vi "helicopter.vi"() -> ()   [LabVIEW 2017]
uses:
  controls/state.ctl
  controls/arrays and heights.ctl
  controls/scores.ctl
  <vilib>/sound2/lvsound2.llb/Sound Output Task ID.ctl
  <vilib>/sound2/lvsound2.llb/Sound Output Set Volume (Single).vi
panel:
  out "Waveform Chart":waveform(dbl)[](graph)=[{"t0"=timestamp(75 s since 1904-01-01), "dt"=1.0, "Y"=[90.36613236635097, 90.06036176170126, 89.42608442122003, 89.31247150775786, 88.85183588729195, 88.07425750121689, 88.69261658515198, 87.86425557558843, 88.68598594735637, 89.37218640366484, 88.87909011717896, 89.2723214289112, 89.37198808916769, 89.3075761436066, 89.59339067781413, 89.09888409349647, 89.89015333376268, 89.02148210217948, 89.47099401182557, 89.25048133248812, 89.38897358327958, 89.77746190833348, 90.53755429906346, 91.28574771023173, 90.94907051126542, 90.31859843418972, 90.86724841965984, 90.63431666280458, 91.36203841742443, 92.04622343431689, 91.2238317034208, 90.39079136550929, 89.84037866388954, 89.6430353390771, 90.19775011068187, 89.34296034585601, 88.87882107659819, 88.68974069015621, 89.40076042601159, 88.75168446743764, 87.95702372899578, 88.65736922287022, 87.90799712470135, 87.54405824486757, 87.74580039145059, 87.72021014407412, 87.91110658053051, 88.72125981331965, 88.50217712958094, 88.66901306015122, 88.44710332072938, 89.2439046034086, 89.44541276476619, 89.49348158640845, 90.23930384605846, 90.77006534815207, 91.56141906157212, 92.1965278095345, 91.61779502995512, 91.68953912575036, 91.7353123580429, 91.13420107041388, 91.29336740149286, 91.62246065547052, 92.32580838508346, 92.94681638984402, 93.63800419438708, 94.43512822801334, 95.09729030042807, 94.89218320830427, 95.29402122869416, 95.18981755244249, 94.53360430397686, 94.27656624709857, 94.95521955315563, 95.75593296599362, 95.13068608073014, 95.87345050233536, 96.41159434256669, 97.01259955208491, 96.59292222657096, 95.89637511486526, 96.58985501237102, 97.18611274172392, 97.70234591984999, 97.33615669802494, 96.72130798541049, 97.44479281384942, 97.84458360370694, 96.99411772170845, 97.83904016371078, 98.54327276615516, 98.84951280333539, 99.26520954670279, 99.7106233231448, 98.89367163173466, 98.55486364541227, 98.33140165697876, 97.47445939153363, 96.91169513152757, 96.77239204274291]}, {"t0"=timestamp(0 s since 1904-01-01), "dt"=1.0, "Y"=[50.0, 50.0, 50.0, 50.0, 50.0, 50.0, 50.0, 50.0, 50.0, 50.0, 50.0, 50.0, 50.0, 50.0, 50.0, 50.0, 50.0, 50.0, 50.0, 50.0, 50.0, 50.0, 50.0, 50.0, 50.0, 50.0, 50.0, 50.0, 50.0, 50.0, 50.0, 50.0, 50.0, 50.0, 50.0, 50.0, 50.0, 49.963212500000004, 49.901900000000005, 49.81606250000001, 49.70570000000001, 49.57081250000001, 49.41140000000001, 49.22746250000001, 49.01900000000001, 48.78601250000001, 48.528500000000015, 48.246462500000014, 47.939900000000016, 47.60881250000002, 47.25320000000002, 46.873062500000024, 46.47777500000002, 46.07358750000002, 45.66675000000002, 45.26351250000002, 44.87012500000002, 44.49283750000002, 44.13790000000002, 43.81156250000002, 43.52007500000002, 43.269687500000025, 43.066650000000024, 42.917212500000026, 42.827625000000026, 42.804137500000024, 42.85300000000002, 42.98046250000002, 43.192490909090935, 43.48605492424245, 43.861154545454575, 44.3177897727273, 44.85596060606064, 45.475667045454585, 46.176909090909135, 46.95968674242429, 47.82400000000005, 48.76984886363641, 49.79723333333339, 50.90615340909097, 52.096609090909155, 53.368600378787946, 54.72212727272734, 56.15718977272734, 57.67378787878795, 59.26254659090916, 60.91721590909098, 62.6315458333334, 64.39928636363643, 66.21418750000008, 68.06999924242433, 69.96047159090918, 71.87935454545463, 73.8203981060607, 75.77735227272736, 77.74396704545464, 79.7139924242425, 81.68117840909099, 83.63927500000008, 85.58203219696978, 87.50320000000009]}, {"t0"=timestamp(75 s since 1904-01-01), "dt"=1.0, "Y"=[5.832101008474922, 5.159278583421013, 5.801309156356126, 6.28595492791603, 6.165150175868025, 5.391838078029318, 5.660821421593425, 6.290693171535654, 5.486359312466074, 4.980595454428121, 5.743102722515479, 5.30778379381289, 5.55585812403333, 4.705780686732893, 5.2333896609954405, 4.963823736280907, 5.822464417498429, 6.642853398607047, 6.668353285980142, 6.089309556691314, 6.609858622855841, 5.982411212743665, 5.438514421617222, 6.263955715844029, 5.531193565870151, 5.801494600625852, 5.566031242846543, 5.115602472848708, 4.8481344780389595, 5.442184030722513, 5.149905285075606, 5.323279727659692, 5.065894282439003, 5.104924163660315, 4.891177011196872, 4.93812604547638, 5.067990838692791, 4.41324137869173, 3.5767367766417517, 2.792679923924744, 2.4382317997087983, 2.671144146629132, 3.1776714395653554, 3.690271474648958, 3.367994065506265, 3.215178406627257, 3.569049632721444, 3.463406971992561, 3.3200051907081365, 3.725695826201605, 3.0566988241284543, 3.4748166261830487, 2.879357702129107, 3.258851993085851, 2.522144166423153, 3.1542111118236003, 3.5230799629696405, 3.9745896259951596, 4.195366575820299, 4.883766157691795, 4.662673212944459, 5.034075317396015, 5.473994783784907, 4.699819872968005, 4.061002012703361, 3.197689491225556, 2.927623166451658, 3.7805700044544763, 3.210549827499141, 3.411153283350134, 2.6885766219340868, 3.4848113994331325, 3.8765381933384324, 3.565085003146204, 4.2186698007162295, 4.443019252189356, 4.859586669337306, 5.307331570893703, 4.60484270830926, 4.8982383059707155, 4.805761589310327, 4.454111165255858, 5.024113691840286, 4.881538126174325, 5.292346594076474, 5.233885183603672, 5.771407868577864, 5.6442442129488715, 6.45349714065848, 6.326226502898815, 5.886373600897694, 6.685385577016143, 7.325174833405951, 7.254372612866276, 7.680755742430742, 7.701210685658931, 7.8289177080882535, 8.447237862350994, 8.214394126067315, 8.955412687632835, 9.120288920602299]}, {"t0"=timestamp(75 s since 1904-01-01), "dt"=1.0, "Y"=[-150.0, -150.0, -150.0, -150.0, -150.0, -150.0, -150.0, -150.0, -150.0, -150.0, -150.0, -150.0, -150.0, -150.0, -150.0, -150.0, -150.0, -150.0, -150.0, -150.0, -150.0, -150.0, -150.0, -150.0, -150.0, -150.0, -150.0, -150.0, -150.0, -150.0, -150.0, -150.0, -150.0, -150.0, -150.0, -150.0, -150.0, -150.0, -150.0, -150.0, -150.0, -150.0, -150.0, -150.0, -150.0, -150.0, 150.0, 150.0, 150.0, 150.0, 150.0, 150.0, 150.0, 150.0, 150.0, 150.0, 38.0, 38.0, 38.0, 38.0, 38.0, 38.0, 38.0, 38.0, 38.0, 38.0, -38.0, -38.0, -38.0, -38.0, -38.0, -38.0, -38.0, -38.0, -38.0, -38.0, 5.0, 5.0, 5.0, 5.0, 5.0, 5.0, 5.0, 5.0, 5.0, 5.0, -5.0, -5.0, -5.0, -5.0, -5.0, -5.0, -5.0, -5.0, -5.0, -5.0, 9.0, 9.0, 9.0, 9.0, 9.0]}]
  in  "View High Scores":bool
  in  "Music?":bool
  out "Score":dbl=132.0 format="%#.12g"
  in  "Difficulty":enum16{"Easy", "Normal", "Hard"}(ring)=enum."Normal"
  out "Acceleration (m/s^2)":dbl(knob)=-7.385757575757571 scale=-10.0..10.0
  in  "Cancel Button":bool
  in  "Start":bool
  out "Fuel (L)":dbl(knob)=150.0 scale=0.0..300.0
  in  "Thrust (m/s^2)":dbl(slide)=21.212121212121215 scale=0.0..50.0
  in  "Vertical Thrusters!":bool
  out "Large Helicopter Image":u8[][](graph)
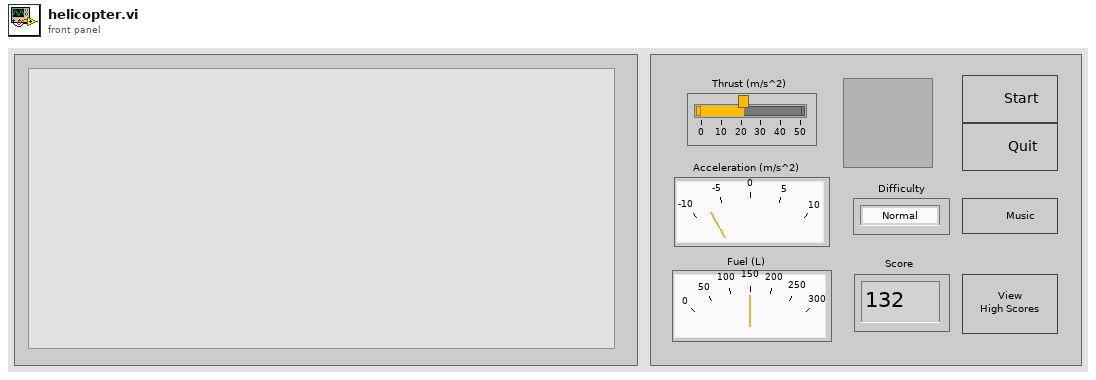
[diagram p1: front panel]
types:
  T1 = typedef "Sound Output Task ID.ctl" = u32
  T2 = typedef "arrays and heights.ctl" = cluster{"Score Array":T3[], "Lowest high score":dbl, "Score":dbl, "Ceiling":dbl, "Floor":dbl, "Ceiling Array":dbl[], "Floor array":dbl[], "Helicopter height":dbl, "Helicopter array":dbl[], "Fuel":dbl, "Fuel array":dbl[], "fuel counter":i32, "obstacle counter":i32, "Obstacle array":dbl[], "helicopter v_0":dbl, "helicopter a_0":dbl, "Obstacle height":dbl}
  T3 = typedef "scores.ctl" = cluster{"Score":dbl, "Name":string, "Date":string}
  T4 = typedef "state.ctl" = enum16{"Wait", "Init", "Run", "Death", "Write High Score", "View High Scores", "Difficulty", "Stop"}
  T5 = typedef "game parameters.ctl" = cluster{"Upper Limit (m)":dbl, "Lower Limit (m)":dbl, "Obstacle time":dbl, "Obstacle length":dbl, "fuel decrement":dbl, "Fuel time":dbl, "fuel amount":dbl, "Fuel range":i32, "Death range":i32, "Terrain slope":dbl, "Speed (km/hr)":dbl, "Time step (ms)":u32, "Gravity":dbl, "Date":string, "High scores path":path, "Difficulty":enum16{"Easy", "Normal", "Hard"}, "Headstart":u32}
  T6 = typedef "Sound Paths.ctl" = cluster{"Crash sound path":path, "Music path":path, "Thrust sound path":path, "High score sound path":path}
  T7 = typedef "image arrays.ctl" = cluster{"Helicopter image":u8[][], "Flame image":u8[][], "Large image":u8[][]}
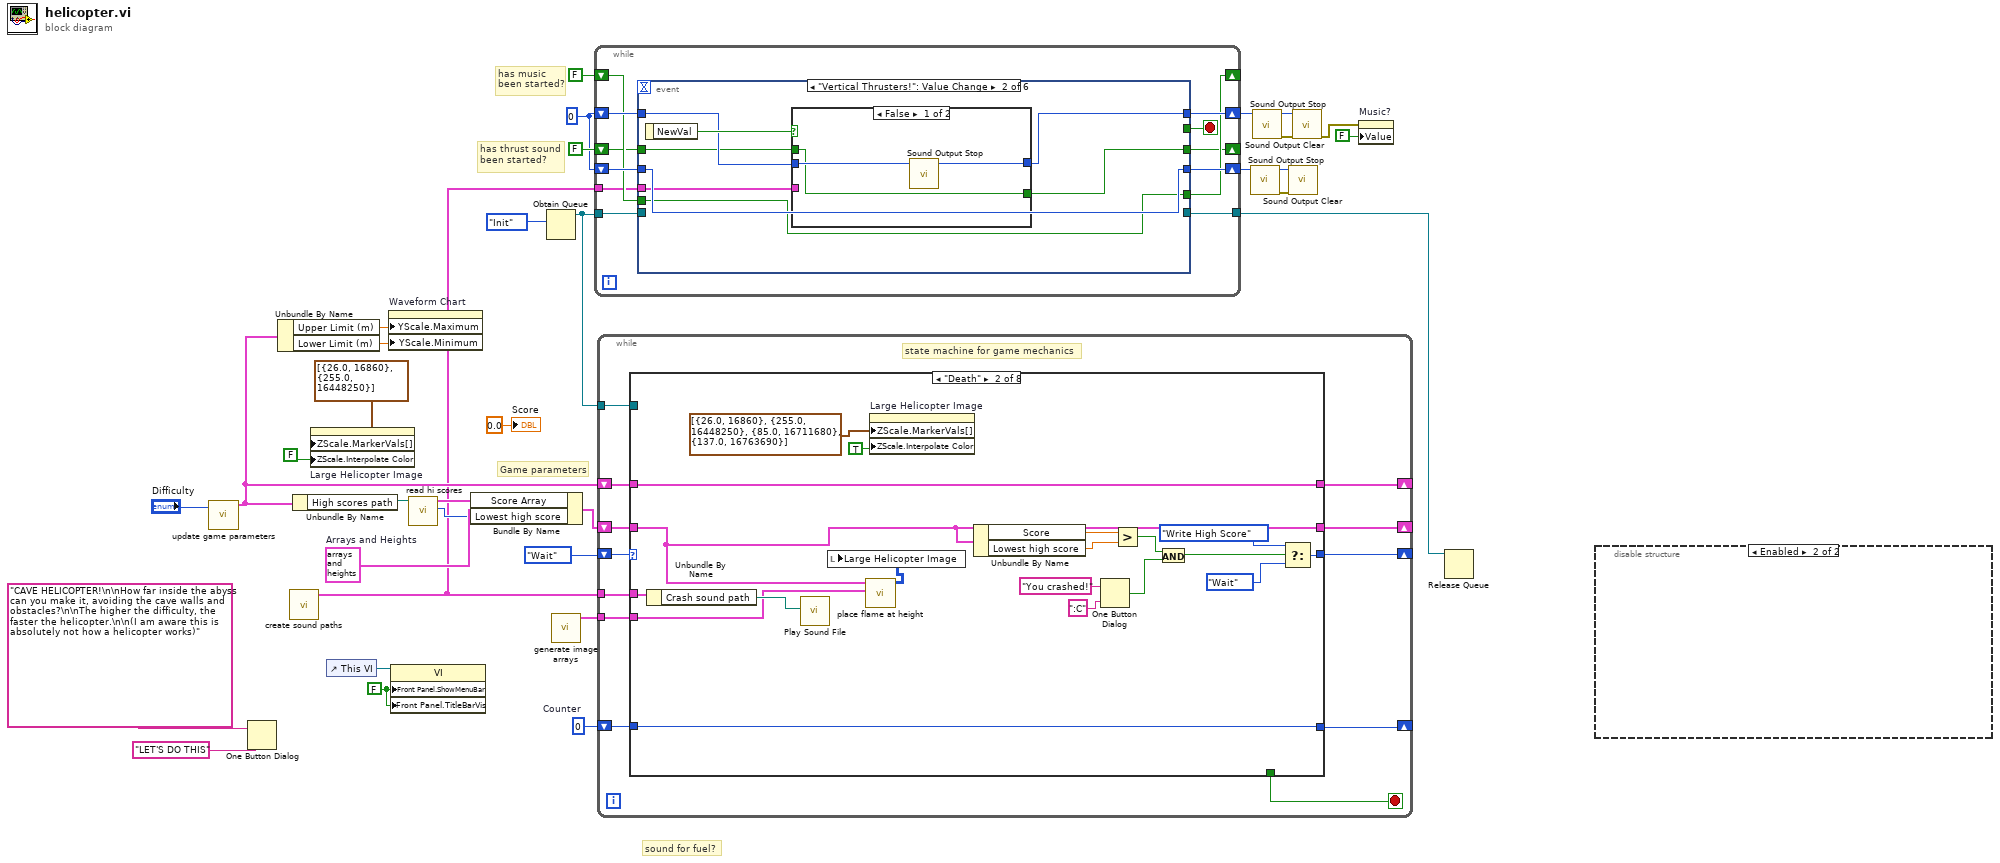
[diagram p0: block diagram]
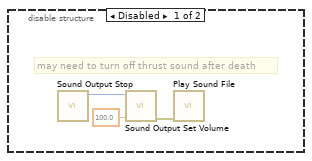
[diagram p2: hidden frame]
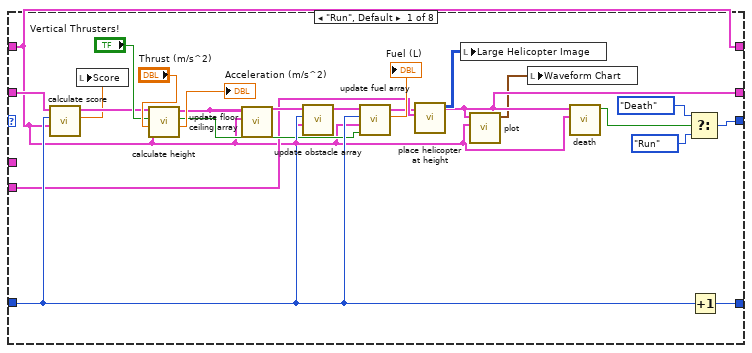
[diagram p3: hidden frame]
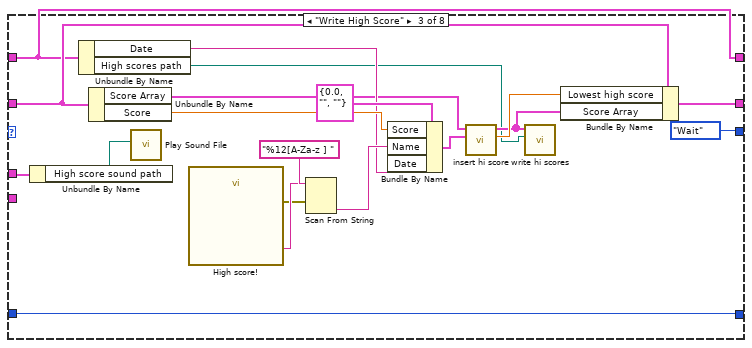
[diagram p4: hidden frame]
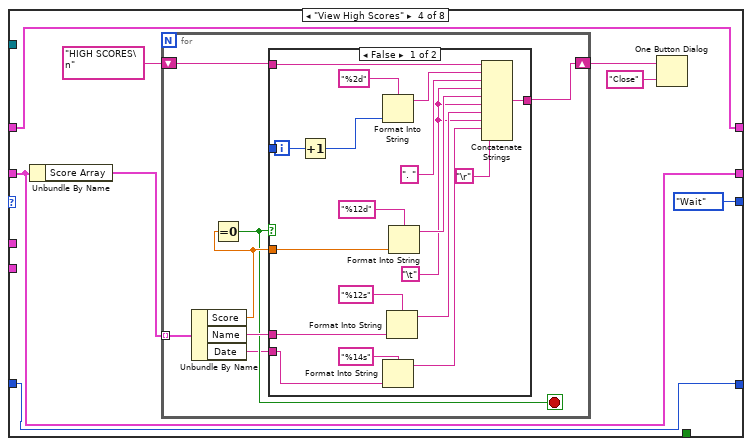
[diagram p5: hidden frame]
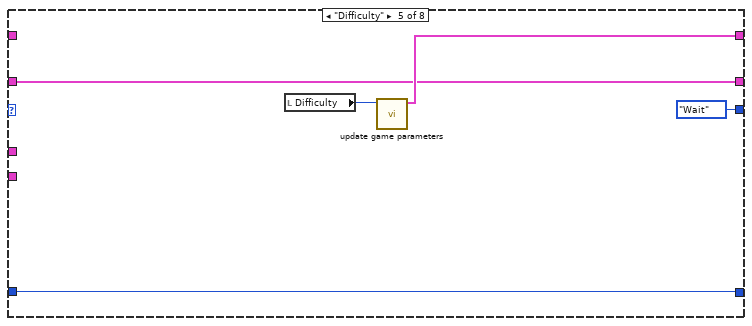
[diagram p7: hidden frame]
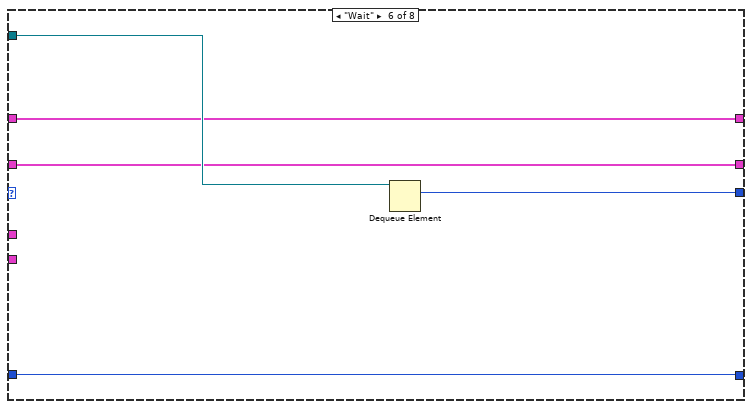
[diagram p8: hidden frame]
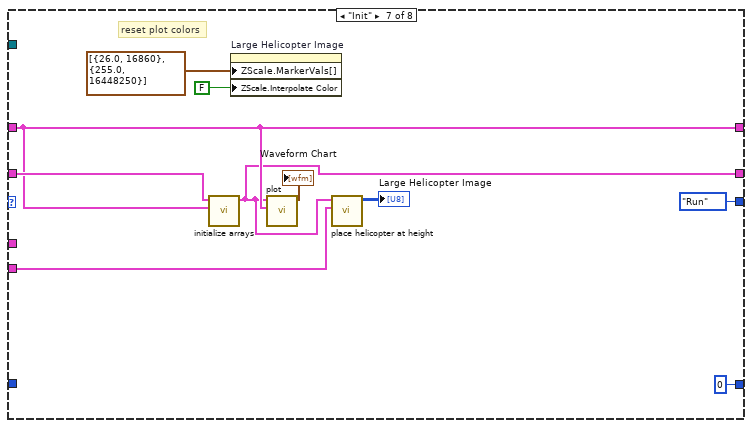
[diagram p9: hidden frame]
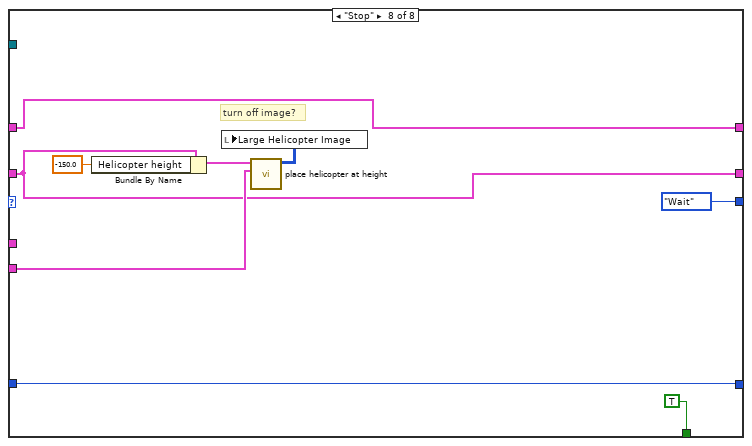
[diagram p10: hidden frame]
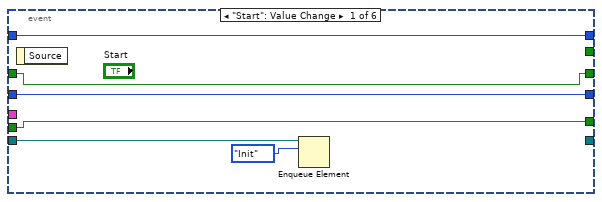
[diagram p11: hidden frame]
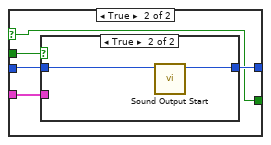
[diagram p12: hidden frame]
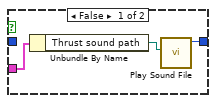
[diagram p13: hidden frame]
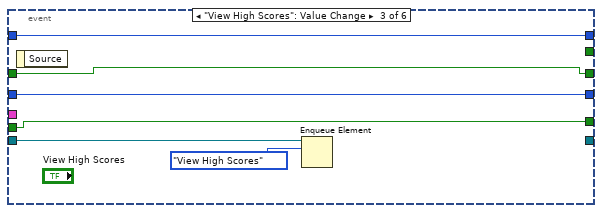
[diagram p14: hidden frame]
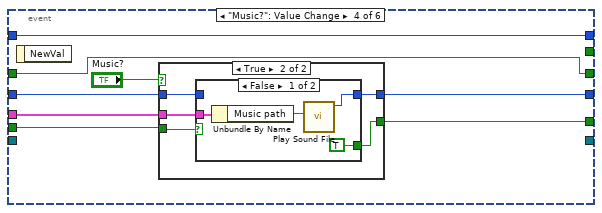
[diagram p15: hidden frame]
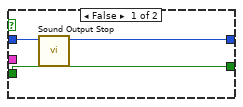
[diagram p16: hidden frame]
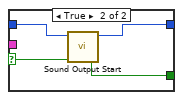
[diagram p17: hidden frame]
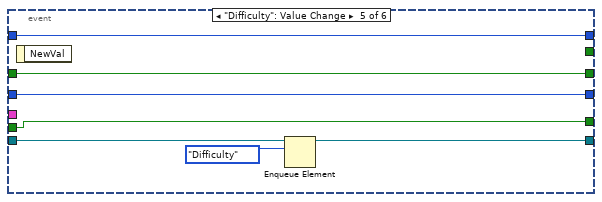
[diagram p18: hidden frame]
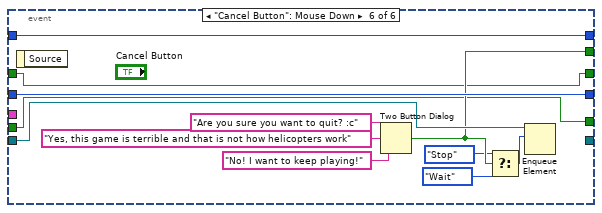
[diagram p19: hidden frame]
diagram:
  w9 = T1 0 ("task ID")
  w22 = T2 {"Score Array"=[], "Lowest high score"=0.0, "Score"=0.0, "Ceiling"=0.0, "Floor"=0.0, "Ceiling Array"=[], "Floor array"=[], "Helicopter height"=0.0, "Helicopter array"=[], "Fuel"=300.0, "Fuel array"=[], "fuel counter"=0, "obstacle counter"=0, "Obstacle array"=[], "helicopter v_0"=0.0, "helicopter a_0"=0.0, "Obstacle height"=300.0}  # Arrays and Heights
  w23 = 0  # Counter
  w33 = FALSE ("Front Panel Window:Show Menu Bar")
  # "has thrust sound\nbeen started?"
  # "has music\nbeen started?"
  # "sound for fuel?"
  # "Game parameters"
  n1 = call "update game parameters.vi"("Difficulty"="Difficulty") -> ("Game Parameters"=w17:T5)  [unwired: 10 in]
  n2 = One Button Dialog(message="CAVE HELICOPTER!\n\nHow far inside the abyss can you make it, avoiding the cave walls and obstacles?\n\nThe higher the difficulty, the faster the helicopter.\n\n(I am aware this is absolutely not how a helicopter works)", button name ("OK")="LET'S DO THIS") -> ()  [unwired: 1 out]
  n3 = Unbundle By Name(w17) -> ("Upper Limit (m)"=w27:dbl, "Lower Limit (m)"=w26:dbl)
  n4 = call "create sound paths.vi"() -> ("Sound Paths"=w11:T6)  [unwired: 11 in]
  n5 = Unbundle By Name(w17) -> ("High scores path"=w16:path)
  n6 = property on="Large Helicopter Image" class="IntGraph (strict)"("ZScale.MarkerVals[]"=cluster{dbl, u32}[] [{26.0, 16860}, {255.0, 16448250}] ("Z Scale.Marker Values[]"), "ZScale.Interpolate Color"=FALSE ("Z Scale.Interpolate Color")) -> ()  [unwired: 2 in, 2 out]
  n7 = control-ref of="This VI"() -> (w34:refnum<vi>)
  n8 = property on="Waveform Chart" class="WFChart (strict)"("YScale.Maximum"=w27, "YScale.Minimum"=w26) -> ()  [unwired: 2 in, 2 out]
  n9 = property class="VI"(reference=w34, "Front Panel.ShowMenuBar"=w33, "Front Panel.TitleBarVis"=w33) -> ()  [unwired: 1 in, 2 out]
  n10 = call "read hi scores.vi"("file path (dialog if empty)"=w16) -> ("Lowest Score"=w14:i64, "Score Array Out"=w15:T3[])  [unwired: 8 in, 1 out]
  n11 = Bundle By Name(cluster=w22, "Score Array"=w15, "Lowest high score"=w14) -> (w18:T2)
  n12 = Obtain Queue(element data type=state."Init" ("State")) -> (queue out=w20:refnum<queue>)  [unwired: 4 in, 2 out]
  n13 = call "generate image arrays.vi"() -> ("Image Arrays"=w21:T7)  [unwired: 11 in]
  n14 = while {
    shift-right: [w45] -> w5
    shift-left: w9 -> [w46]
    tunnel: w20 -> [w43]
    shift-right: [w41] -> w3
    shift-left: w9 -> [w42]
    tunnel: [w40] -> w13
    shift-right: [w38] -> _
    shift-left: FALSE -> [w39]
    tunnel: w11 -> [w37]
    shift-right: [w35] -> _
    shift-left: FALSE -> [w36]
    stop <- w44 stop-if-true
    n15 = event shown="[1] \"Vertical Thrusters!\": Value Change" {
      selector: _ -> [_ _ _ _ _ _]
      dyn-events: _ -> [_ _ _ _ _ _]
      timeout: _ -> [_ _ _ _ _ _]
      tunnel: [_ _ _ _ _ w115] -> w44
      tunnel: w46 -> [w52 w57 w79 w87 w109 w121]
      tunnel: [w52 w57 w79 w86 w109 w121] -> w45
      tunnel: w43 -> [w50 _ w78 _ w108 w116]
      tunnel: w42 -> [w51 w59 w77 w85 w106 w117]
      tunnel: [w51 w58 w77 w85 w106 w117] -> w41
      tunnel: [_ _ _ _ w105 _] -> w40
      tunnel: w39 -> [w48 w53 w74 w83 w103 w110]
      tunnel: [w48 w53 w74 w82 w103 w110] -> w38
      tunnel: w37 -> [_ w55 _ w81 _ _]
      tunnel: w36 -> [w47 w56 w75 w80 w104 w111]
      tunnel: [w47 w54 w75 w80 w104 w111] -> w35
      event "Start": Value Change {
        n16 = event-data() -> ()  [unwired: 1 in, 1 out]
        n17 = Enqueue Element(queue=w50, element=state."Init") -> ()  [unwired: 2 in, 3 out]
      }
      event "Vertical Thrusters!": Value Change {
        n18 = event-data() -> ("NewVal"=w60:bool)  [unwired: 1 in]
        n19 = case shown="False" w60 {
          selector: w60 -> [_ w64]
          tunnel: [w63 w68] -> w58
          tunnel: w59 -> [w62 w67]
          tunnel: w56 -> [w61 w65]
          tunnel: w55 -> [_ w66]
          tunnel: [w61 w64] -> w54
          frame False {
            n20 = call <vilib>:"Sound Output Stop.vi"("task ID"=w62) -> ("task ID out"=w63:T1)  [unwired: 9 in, 1 out]
          }
          frame True {
            n21 = case shown="True" w65 {
              tunnel: [w69 w73] -> w68
              tunnel: w67 -> [_ w72]
              tunnel: w66 -> [w70 _]
              frame False {
                n22 = Unbundle By Name(w70) -> ("Thrust sound path"=w71:path)
                n23 = call <vilib>:"Play Sound File.vi"("path"=w71) -> ("task ID"=w69:T1)  [unwired: 9 in, 1 out]
              }
              frame True {
                n24 = call <vilib>:"Sound Output Start.vi"("task ID"=w72) -> ("task ID out"=w73:T1)  [unwired: 9 in, 1 out]
              }
            }
          }
        }
      }
      event "View High Scores": Value Change {
        n25 = event-data() -> ()  [unwired: 1 in, 1 out]
        n26 = Enqueue Element(queue=w78, element=state."View High Scores") -> ()  [unwired: 2 in, 3 out]
      }
      event "Music?": Value Change {
        n27 = event-data() -> ()  [unwired: 1 in, 1 out]
        n28 = case shown="True" "Music?" {
          tunnel: w87 -> [w90 w94]
          tunnel: [w89 w95] -> w86
          tunnel: w83 -> [w88 w93]
          tunnel: [w88 w92] -> w82
          tunnel: w81 -> [_ w91]
          frame False {
            n29 = call <vilib>:"Sound Output Stop.vi"("task ID"=w90) -> ("task ID out"=w89:T1)  [unwired: 9 in, 1 out]
          }
          frame True {
            n30 = case shown="False" w93 {
              selector: w93 -> [_ w100]
              tunnel: [w98 w102] -> w95
              tunnel: w94 -> [_ w101]
              tunnel: [TRUE w100] -> w92
              tunnel: w91 -> [w96 _]
              frame False {
                n31 = Unbundle By Name(w96) -> ("Music path"=w99:path)
                n32 = call <vilib>:"Play Sound File.vi"("path"=w99) -> ("task ID"=w98:T1)  [unwired: 9 in, 1 out]
              }
              frame True {
                n33 = call <vilib>:"Sound Output Start.vi"("task ID"=w101) -> ("task ID out"=w102:T1)  [unwired: 9 in, 1 out]
              }
            }
          }
        }
      }
      event "Difficulty": Value Change {
        n34 = event-data() -> ()  [unwired: 1 in, 1 out]
        n35 = Enqueue Element(queue=w108, element=state."Difficulty") -> (queue out=w105:refnum<queue>)  [unwired: 2 in, 2 out]
      }
      event "Cancel Button": Mouse Down {
        n36 = event-data() -> ()  [unwired: 1 in, 1 out]
        n37 = Two Button Dialog(message="Are you sure you want to quit? :c", 1:"No! I want to keep playing!" ("F button name (\"Cancel\")"), 2:"Yes, this game is terrible and that is not how helicopters work" ("T button name (\"OK\")")) -> (T button?=w115:bool)
        n38 = Select(t=state."Stop" ("State"), s=w115, f=state."Wait" ("State")) -> (s? t:f=w113:T4)
        n39 = Enqueue Element(queue=w116, element=w113) -> ()  [unwired: 2 in, 3 out]
      }
    }
  }
  n40 = while {
    shift-right: [w133] -> _
    shift-left: state."Wait" ("State") -> [w132]
    tunnel: w20 -> [w131]
    shift-right: [w129] -> _
    shift-left: w23 -> [w130]
    shift-right: [w128] -> _
    shift-left: w18 -> [w126]
    tunnel: w21 -> [w127]
    tunnel: w11 -> [w124]
    shift-right: [w122] -> _
    shift-left: w17 -> [w123]
    stop <- w125 stop-if-true
    # "state machine for game mechanics"
    n41 = case shown="\"Death\"" w132 {
      tunnel: [w153 w166 state."Wait" ("State") state."Wait" ("State") state."Wait" ("State") w238 state."Run" ("State") state."Wait" ("State")] -> w133
      tunnel: w131 -> [_ _ _ _ _ w237 _ _]
      tunnel: w130 -> [w145 w174 w175 w194 w229 w236 _ w250]
      tunnel: [w151 w174 w175 w194 w229 w236 0 w250] -> w129
      tunnel: [w139 w159 w181 w195 w230 w235 w239 w252] -> w128
      tunnel: w127 -> [w141 w160 _ _ _ _ w242 w253]
      tunnel: w126 -> [w137 w159 w182 w195 w230 w235 w241 w252]
      tunnel: [_ _ _ _ _ _ _ TRUE] -> w125
      tunnel: w124 -> [_ w169 w189 _ _ _ _ _]
      tunnel: w123 -> [w134 w156 w176 w196 _ w234 w240 w249]
      tunnel: [w134 w156 w176 w196 w231 w234 w240 w249] -> w122
      frame "Run", Default {
        n42 = call "calculate score.vi"("Game Parameters"=w134, "loop count"=w145, "Arrays and Heights"=w137) -> ("Score"=w135:dbl, "Arrays and Heights"=w136:T2)  [unwired: 7 in]
        n43 = local write "Score"(w135) -> ()
        n44 = call "calculate height.vi"("Game Parameters"=w134, "Thrust (m/s^2)"="Thrust (m/s^2)", "Thrusters on?"="Vertical Thrusters!", "Arrays and Heights"=w136) -> ("Acceleration (m/s^2)"=→"Acceleration (m/s^2)":dbl, "Decrement fuel?"=w144:bool, "Arrays and Heights"=w140:T2)  [unwired: 5 in]
        n45 = call "update floor ceiling array.vi"("Game Parameters"=w134, "Arrays and Heights"=w140) -> ("Arrays and Heights"=w147:T2)  [unwired: 9 in]
        n46 = call "update obstacle array.vi"("Game Parameters"=w134, "loop counter"=w145, "Arrays and Heights"=w147) -> ("Arrays and heights"=w146:T2)  [unwired: 8 in]
        n47 = call "update fuel array.vi"("Decrement fuel?"=w144, "Game Parameters"=w134, "step count"=w145, "Arrays and values"=w146) -> ("Fuel (L)"=→"Fuel (L)":dbl, "Arrays and Heights"=w139:T2)  [unwired: 6 in]
        n48 = call "place helicopter at height.vi"("Image Arrays"=w141, "Arrays and Heights"=w140) -> ("Large image"=w142:u8[][])  [unwired: 9 in]
        n49 = local write "Large Helicopter Image"(w142) -> ()
        n50 = call "plot.vi"("Game Parameters"=w134, "Arrays and Heights"=w139) -> ("Waveform Chart"=w138:waveform(dbl)[])  [unwired: 9 in]
        n51 = local write "Waveform Chart"(w138) -> ()
        n52 = call "death.vi"("Game Parameters"=w134, "Arrays and Heights"=w139) -> ("Death?"=w152:bool)  [unwired: 9 in]
        n53 = Select(t=state."Death" ("State"), s=w152, f=state."Run" ("State")) -> (s? t:f=w153:T4)
        n54 = Increment(x=w145) -> (x+1=w151:i32)
      }
      frame "Death" {
        n55 = Unbundle By Name(w169) -> ("Crash sound path"=w168:path)
        n56 = call <vilib>:"Play Sound File.vi"("path"=w168) -> ()  [unwired: 9 in, 2 out]
        n57 = call "place flame at height.vi"("Image Arrays"=w160, "Arrays and Heights"=w159) -> ("Large image"=w161:u8[][])  [unwired: 9 in]
        n58 = local write "Large Helicopter Image"(w161) -> ()
        n59 = property on="Large Helicopter Image" class="IntGraph (strict)"("ZScale.MarkerVals[]"=cluster{dbl, u32}[] [{26.0, 16860}, {255.0, 16448250}, {85.0, 16711680}, {137.0, 16763690}] ("Z Scale.Marker Values[]"), "ZScale.Interpolate Color"=TRUE ("Z Scale.Interpolate Color")) -> ()  [unwired: 2 in, 2 out]
        n60 = Unbundle By Name(w159) -> ("Score"=w158:dbl, "Lowest high score"=w157:dbl)
        n61 = One Button Dialog(message="You crashed!", button name ("OK")=":C" ("message")) -> (true=w162:bool)
        n62 = Greater?(x=w158, y=w157) -> (0:w164:bool)
        n63 = And(x=w164, y=w162) -> (x .and. y?=w163:bool)
        n64 = Select(t=state."Write High Score", s=w163, f=state."Wait" ("State")) -> (s? t:f=w166:T4)
      }
      frame "Write High Score" {
        n65 = Unbundle By Name(w189) -> ("High score sound path"=w188:path)
        n66 = Unbundle By Name(w176) -> ("Date"=w184:string, "High scores path"=w177:path)
        n67 = Unbundle By Name(w182) -> ("Score Array"=w183:T3[], "Score"=w185:dbl)
        n68 = call <vilib>:"Play Sound File.vi"("path"=w188) -> ()  [unwired: 9 in, 2 out]
        n69 = call "High score!"() -> ("Name"=w190:string, "error out"=w187:errorcluster)  [unwired: 17 in, 1 out]
        n70 = Scan From String(format string="%12[A-Za-z ] ", input string=w190, error in=w187) -> (output 1=w193:string)  [unwired: 2 in, 3 out]
        n71 = Bundle By Name(cluster=T3 {"Score"=0.0, "Name"="", "Date"=""} ("Scores"), "Score"=w185, "Name"=w193, "Date"=w184) -> (w186:T3)
        n72 = call "insert hi score.vi"("Score to Insert"=w186, "Score Array In"=w183) -> ("Lowest Score Out"=w180:dbl, "Score Array Out"=w179:T3[])  [unwired: 7 in, 1 out]
        n73 = call "write hi scores.vi"("file path (dialog if empty)"=w177, "Score Array In"=w179) -> ()  [unwired: 9 in, 1 out]
        n74 = Bundle By Name(cluster=w182, "Lowest high score"=w180, "Score Array"=w179) -> (w181:T2)
      }
      frame "View High Scores" {
        n75 = Unbundle By Name(w195) -> ("Score Array"=w197:T3[])
        n76 = for {
          tunnel: w197 -> [w209] mode=indexing
          shift-right: [w207] -> w199
          shift-left: "HIGH SCORES\n" -> [w206]
          i -> [w208]
          stop <- w203 stop-if-true
          n77 = Unbundle By Name(w209) -> ("Score"=w204:dbl, "Name"=w205:string, "Date"=w202:string)
          n78 = Equal To 0?(x=w204) -> (x = 0?=w203:bool)
          n79 = case shown="False" w203 {
            tunnel: w208 -> [w227 _]
            tunnel: [w224 w228] -> w207
            tunnel: w206 -> [w219 w228]
            tunnel: w205 -> [w216 _]
            tunnel: w204 -> [w211 _]
            tunnel: w202 -> [w210 _]
            frame False {
              w214 = "\t"
              n80 = Increment(x=w227) -> (x+1=w223:i32)
              n81 = Format Into String(format string="%2d", w223) -> (resulting string=w220:string)  [unwired: 2 in, 1 out]
              n82 = Format Into String(format string="%14s", w210) -> (resulting string=w213:string)  [unwired: 2 in, 1 out]
              n83 = Format Into String(format string="%12s", w216) -> (resulting string=w218:string)  [unwired: 2 in, 1 out]
              n84 = Format Into String(format string="%12d", w211) -> (resulting string=w225:string)  [unwired: 2 in, 1 out]
              n85 = Concatenate Strings(w219, w220, ". " ("string"), w214, w225, w214, w218, w214, w213, "\r") -> (w224:string)
            }
            frame True {
            }
          }
        }
        n86 = One Button Dialog(message=w199, button name ("OK")="Close") -> ()  [unwired: 1 out]
      }
      frame "Difficulty" {
        n87 = local read "Difficulty"() -> (w232:enum16{"Easy", "Normal", "Hard"})
        n88 = call "update game parameters.vi"("Difficulty"=w232) -> ("Game Parameters"=w231:T5)  [unwired: 10 in]
      }
      frame "Wait" {
        n89 = Dequeue Element(queue=w237) -> (element=w238:T4)  [unwired: 2 in, 3 out]
      }
      frame "Init" {
        # "reset plot colors"
        n90 = call "initialize arrays.vi"("Game Parameters"=w240, "Arrays and Heights"=w241) -> ("Arrays and values"=w239:T2)  [unwired: 9 in]
        n91 = property on="Large Helicopter Image" class="IntGraph (strict)"("ZScale.MarkerVals[]"=cluster{dbl, u32}[] [{26.0, 16860}, {255.0, 16448250}] ("Z Scale.Marker Values[]"), "ZScale.Interpolate Color"=FALSE ("Z Scale.Interpolate Color")) -> ()  [unwired: 2 in, 2 out]
        n92 = call "plot.vi"("Game Parameters"=w240, "Arrays and Heights"=w239) -> ("Waveform Chart"=→"Waveform Chart":waveform(dbl)[])  [unwired: 9 in]
        n93 = call "place helicopter at height.vi"("Image Arrays"=w242, "Arrays and Heights"=w239) -> ("Large image"=→"Large Helicopter Image":u8[][])  [unwired: 9 in]
      }
      frame "Stop" {
        # "turn off image?"
        n94 = Bundle By Name(cluster=w252, "Helicopter height"=-150.0) -> (w254:T2)
        n95 = call "place helicopter at height.vi"("Image Arrays"=w253, "Arrays and Heights"=w254) -> ("Large image"=w256:u8[][])  [unwired: 9 in]
        n96 = local write "Large Helicopter Image"(w256) -> ()
      }
    }
  }
  n97 = call <vilib>:"Sound Output Stop.vi"("task ID"=w5) -> ("error out"=w6:errorcluster, "task ID out"=w4:T1)  [unwired: 9 in]
  n98 = call <vilib>:"Sound Output Stop.vi"("task ID"=w3) -> ("error out"=w7:errorcluster, "task ID out"=w2:T1)  [unwired: 9 in]
  n99 = call <vilib>:"Sound Output Clear.vi"("error in (no error)"=w6, "task ID"=w4) -> ()  [unwired: 9 in, 1 out]
  n100 = call <vilib>:"Sound Output Clear.vi"("error in (no error)"=w7, "task ID"=w2) -> ("error out"=w1:errorcluster)  [unwired: 9 in]
  n101 = property on="Music?" class="Bool (strict)"(error in=w1, "Value"=FALSE ("Music?")) -> ()  [unwired: 1 in, 2 out]
  n102 = Release Queue(queue=w13) -> ()  [unwired: 2 in, 3 out]
  n103 = disable-structure shown="Enabled" {
    frame Disabled {
      # "may need to turn off thrust sound after death"
      n104 = call <vilib>:"Sound Output Stop.vi"() -> ("task ID out"=w260:T1)  [unwired: 10 in, 1 out]
      n105 = call-poly <vilib>:"Sound Output Set Volume.vi"("volume"=100.0, "task ID"=w260) -> ("error out"=w259:errorcluster)  [unwired: 8 in, 1 out]
      n106 = call <vilib>:"Play Sound File.vi"("error in (no error)"=w259) -> ()  [unwired: 9 in, 2 out]
    }
    frame Enabled {
    }
  }
  "Score" <- 0.0 ("Score")
